vi "Var_Axis (SubVI).vi"(10 "Value":u16[](array[numeric]), 11 "Value 2":u16[](array[numeric])) -> (2 "Value 3":u16[](array[numeric]), 3 "Array":i32[](array[numeric]))   [LabVIEW 2020]
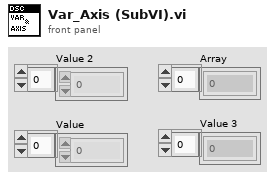
[diagram p1: front panel]
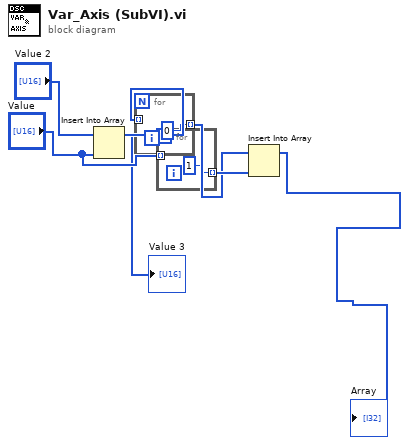
[diagram p0: block diagram]
diagram:
  n1 = Insert Into Array(array="Value 2", new element="Value") -> (→"Value 3":u16[])  [unwired: 1 in]
  n2 = for {
    tunnel: "Value 2" -> [_] mode=indexing
    tunnel: [0 ("index")] -> w4 mode=indexing
  }
  n3 = for {
    tunnel: "Value" -> [_] mode=indexing
    tunnel: [1 ("index")] -> w5 mode=indexing
  }
  n4 = Insert Into Array(array=w4, new element=w5) -> (→"Array":i32[])  [unwired: 1 in]
